vi "Test communication.vi"() -> ()   [LabVIEW 2019, in "CommandResponse communication.lvlib"]
uses:
  CommandResponse communication.lvlib
  NS slave_class/NS slave.lvclass
  NS master_class/NS master.lvclass
panel:
  out "timed out?":bool
  out "slave-last recieved data":variant
  out "slave.last recieved msg":string
  out "master.recieved data":cdb[](array[numeric])
  in  "master.data":cdb
  in  "master.message":string
  in  "send msg":bool
  in  "Stop Button":bool
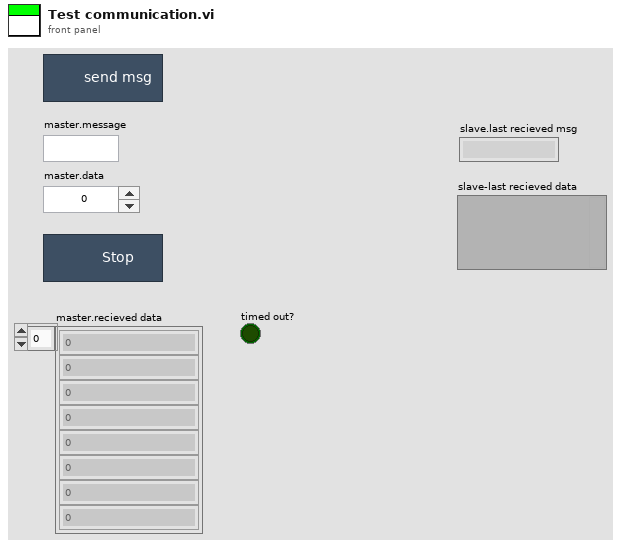
[diagram p1: front panel]
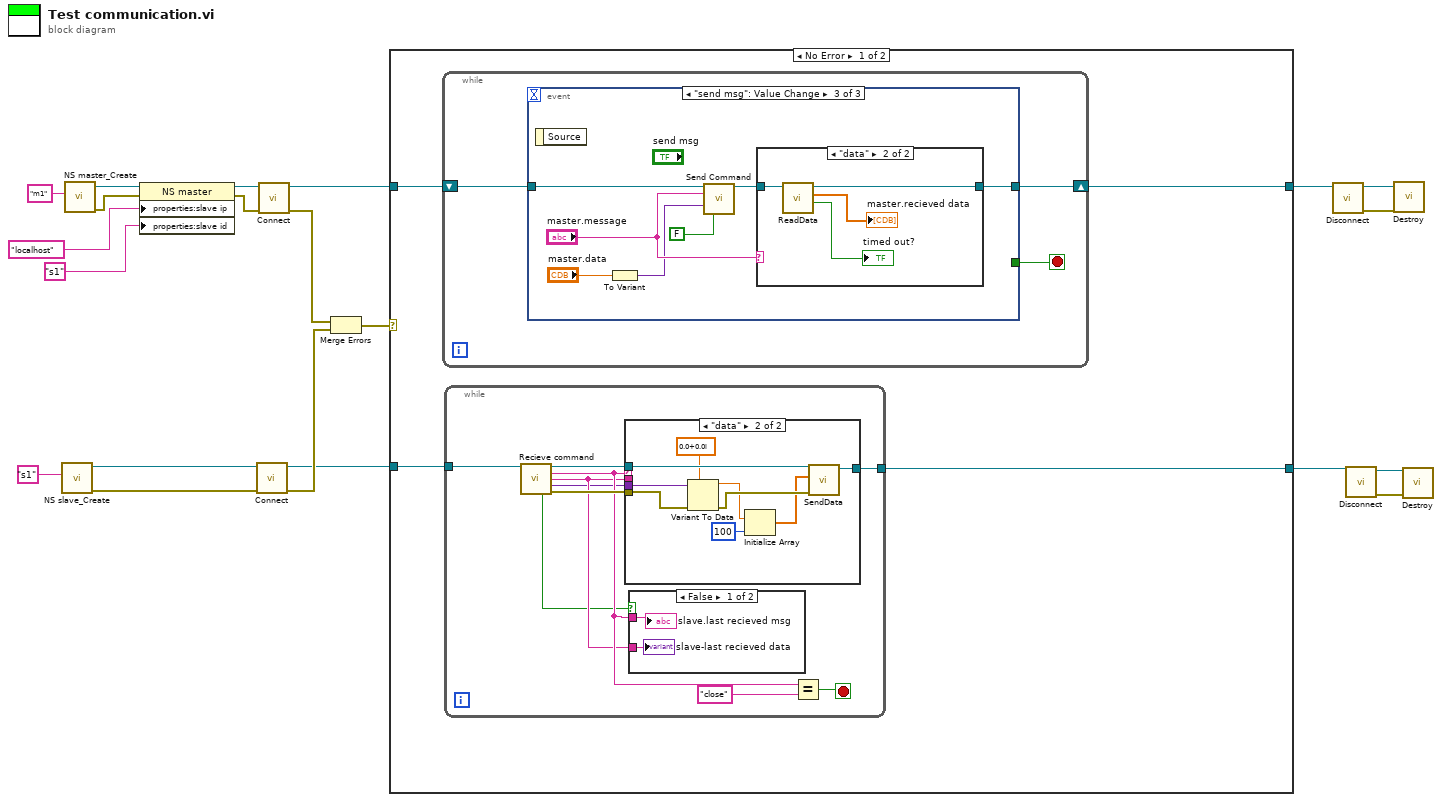
[diagram p0: block diagram]
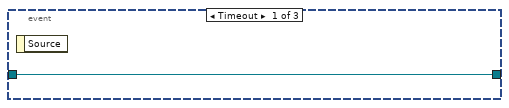
[diagram p4: hidden frame]
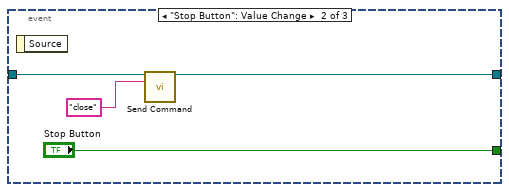
[diagram p5: hidden frame]
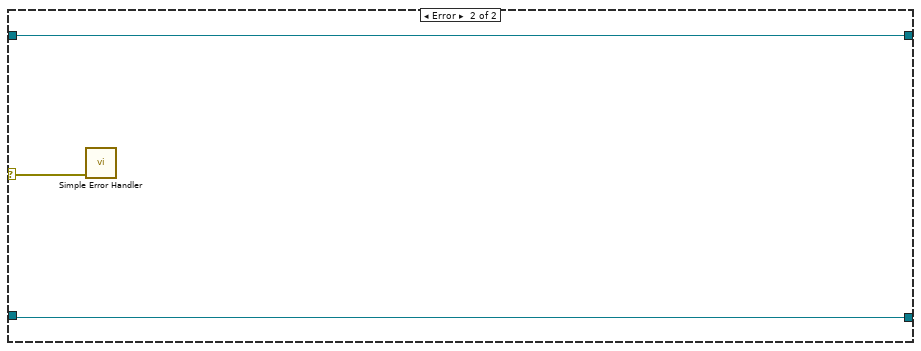
[diagram p7: hidden frame]
diagram:
  n1 = call "NS slave_Create.vi"("ID"="s1") -> ("error out"=w18:errorcluster, "reference out"=w19:refnum<class "NS slave.lvclass">)  [unwired: 9 in]
  n2 = call "NS master_Create.vi"("ID"="m1") -> ("error out"=w4:errorcluster, "reference out"=w17:refnum<class "NS master.lvclass">)  [unwired: 9 in]
  n3 = property class="NS master"(reference=w17, error in=w4, "properties:slave ip"="localhost" ("Slave IP"), "properties:slave id"="s1" ("ID")) -> (reference out=w5:refnum<class "NS master.lvclass">, error out=w3:errorcluster)
  n4 = call-dynamic "Connect.vi"("error in (no error)"=w18, "reference in"=w19) -> ("error out"=w14:errorcluster, "reference out"=w11:refnum<class "NS slave.lvclass">)  [unwired: 8 in]
  n5 = call-dynamic "Connect.vi"("error in (no error)"=w3, "reference in"=w5) -> ("error out"=w15:errorcluster, "reference out"=w16:refnum<class "NS master.lvclass">)  [unwired: 8 in]
  n6 = Merge Errors(w15, w14) -> (w13:errorcluster)
  n7 = case shown="No Error" w13 {
    selector: w13 -> [_ w68]
    tunnel: w16 -> [w25 w70]
    tunnel: [w24 w70] -> w12
    tunnel: w11 -> [w23 w69]
    tunnel: [w22 w69] -> w10
    frame No Error {
      n8 = while {
        shift-right: [w48] -> w24
        shift-left: w25 -> [w49]
        stop <- w50 stop-if-true
        n9 = event shown="[2] \"send msg\": Value Change" {
          selector: _ -> [_ _ _]
          dyn-events: _ -> [_ _ _]
          timeout: _ -> [_ _ _]
          tunnel: [_ "Stop Button" _] -> w50
          tunnel: w49 -> [w51 w54 w62]
          tunnel: [w51 w52 w60] -> w48
          event Timeout {
            n10 = event-data() -> ()  [unwired: 1 in, 1 out]
          }
          event "Stop Button": Value Change {
            n11 = event-data() -> ()  [unwired: 1 in, 1 out]
            n12 = call-dynamic "Send Command.vi"("reference in"=w54, "message"="close") -> ("reference out"=w52:refnum<class "NS master.lvclass">)  [unwired: 9 in, 4 out]
          }
          event "send msg": Value Change {
            n13 = event-data() -> ()  [unwired: 1 in, 1 out]
            n14 = To Variant(anything="master.data") -> (Variant=w56:variant)
            n15 = call-dynamic "Send Command.vi"("reference in"=w62, "message"="master.message", "data"=w56, "response?"=FALSE) -> ("reference out"=w59:refnum<class "NS master.lvclass">)  [unwired: 7 in, 4 out]
            n16 = case shown="\"data\"" "master.message" {
              tunnel: [w63 w66] -> w60
              tunnel: w59 -> [w63 w67]
              frame "False", Default {
              }
              frame "data" {
                n17 = call-dynamic "ReadData.vi"("reference in"=w67) -> ("timed out?"=→"timed out?":bool, "data"=→"master.recieved data":cdb[], "reference out"=w66:refnum<class "NS master.lvclass">)  [unwired: 7 in, 1 out]
              }
            }
          }
        }
      }
      n18 = while {
        tunnel: w23 -> [w35]
        tunnel: [w30] -> w22
        stop <- w33 stop-if-true
        n19 = call-dynamic "Recieve command.vi"("reference in"=w35) -> ("reference out"=w32:refnum<class "NS slave.lvclass">, "message"=w29:string, "parameters"=w28:string, "data"=w26:variant, "timed out?"=w27:bool, "error out"=w31:errorcluster)  [unwired: 9 in]
        n20 = case shown="\"data\"" w29 {
          tunnel: w28 -> [_ _]
          tunnel: w32 -> [w38 w47]
          tunnel: w31 -> [_ w46]
          tunnel: [w38 w44] -> w30
          tunnel: w26 -> [_ w39]
          frame "False", Default {
          }
          frame "data" {
            n21 = Variant To Data(error in=w46, type=cdb 0.0+0.0i ("data 2"), Variant=w39) -> (data=w40:cdb, error out=w45:errorcluster)
            n22 = Initialize Array(w40, 100 ("dimension size")) -> (w42:cdb[])
            n23 = call-dynamic "SendData.vi"("error in (no error)"=w45, "data"=w42, "reference in"=w47) -> ("reference out"=w44:refnum<class "NS slave.lvclass">)  [unwired: 6 in, 2 out]
          }
        }
        n24 = case shown="False" w27 {
          tunnel: w29 -> [w37 _]
          tunnel: w28 -> [w36 _]
          frame False {
            "slave.last recieved msg" <- w37
            "slave-last recieved data" <- w36
          }
          frame True {
          }
        }
        n25 = Equal?(x=w29, y="close") -> (x = y?=w33:bool)
      }
    }
    frame Error {
      n26 = call <vilib>:"Simple Error Handler.vi"("error in (no error)"=w68) -> ()  [unwired: 4 in, 5 out]
    }
  }
  n27 = call-dynamic "Disconnect.vi"("reference in"=w12) -> ("error out"=w9:errorcluster, "reference out"=w8:refnum<class "NS master.lvclass">)  [unwired: 9 in]
  n28 = call-dynamic "Disconnect.vi"("reference in"=w10) -> ("error out"=w7:errorcluster, "reference out"=w6:refnum<class "NS slave.lvclass">)  [unwired: 9 in]
  n29 = call-dynamic "Destroy.vi"("reference in"=w8, "error in (no error)"=w9) -> ()  [unwired: 16 in, 2 out]
  n30 = call-dynamic "Destroy.vi"("reference in"=w6, "error in (no error)"=w7) -> ()  [unwired: 16 in, 2 out]
